vi "Determine Analog and Digital Values for Channels.vi"(10 "Remaining Time":dbl, 11 "Step Settings":T1) -> (2 "Digital Values to Write":bool[](array[boolean]), 3 "Analog Values to Write":dbl[](array[numeric]))   [LabVIEW 2020, in "Sequencer with Output Values.lvlib" / "Sequencer with Output Values.lvclass"]
uses:
  Sequencer with Output Values.lvclass
  Step Settings.ctl
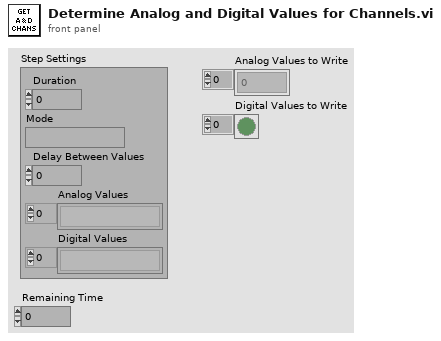
[diagram p1: front panel]
types:
  T1 = typedef "Step Settings.ctl" = cluster{"Duration":dbl, "Mode":string, "Delay Between Values":dbl, "Analog Values":string[], "Digital Values":string[]}
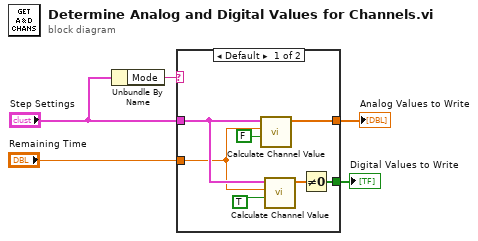
[diagram p0: block diagram]
diagram:
  n1 = Unbundle By Name("Step Settings") -> ("Mode"=w4:string)
  n2 = case shown="Default" w4 {
    tunnel: "Step Settings" -> [w11 _]
    tunnel: "Remaining Time" -> [w10 _]
    tunnel: [w8 _] -> w2
    tunnel: [w6 _] -> w1
    frame Default {
      n3 = call "Calculate Channel Value.vi"("Digital"=FALSE, "Remaining Time"=w10, "Step Settings"=w11) -> ("Values to Write"=w8:dbl[])  [unwired: 8 in]
      n4 = call "Calculate Channel Value.vi"("Digital"=TRUE, "Remaining Time"=w10, "Step Settings"=w11) -> ("Values to Write"=w7:dbl[])  [unwired: 8 in]
      n5 = Not Equal To 0?(x=w7) -> (x != 0?=w6:bool[])
    }
    frame "" {
      # "Don't need to worry about analog or digital channels if mode is empty string"
    }
  }
  "Analog Values to Write" <- w2
  "Digital Values to Write" <- w1
